vi "Aux-Inputs.vi"(8 "error in (no error)":errorcluster, 11 "Node Ptr":T2 format="%.0x") -> (0 "error out":errorcluster)   [LabVIEW 2016, in "DCM System Explorer.lvlib"]
uses:
  DCM System Explorer.lvlib
  <vilib>/NI Veristand/Custom Device API/Custom Device Item Ref.ctl
  <vilib>/Powertrain Controls/Device Drivers/DCM/Rev0/FPGA/Digital Channel.ctl
  Shared/DCM Properties.vi
  <vilib>/NI Veristand/Custom Device API/Get Item Property (String Array).vi
  <vilib>/NI Veristand/Custom Device API/Get Item Property (Double Array).vi
  <vilib>/NI Veristand/Custom Device API/Get Item Property (U16).vi
  Shared/DCM Constants and GUIDs.vi
  <vilib>/NI Veristand/Custom Device API/Set Item Property (String Array).vi
  <vilib>/NI Veristand/Custom Device API/Set Item Property (Double Array).vi
  <vilib>/NI Veristand/Custom Device API/Set Item Property (U16).vi
  <vilib>/NI VeriStand/Custom Device API/Custom Device API.lvlib
  DCM Shared.lvlib
  <vilib>/Powertrain Controls/Device Drivers/DCM/Rev0/FPGA/DCM - FPGA.lvlib
panel:
  in  "Serial Aux In 9-16":T1(ring)
  in  "Serial Aux In 1-8":T1(ring)
  in  "Digital filter [s]":sgl format="%#_2p"
  in  "Filters":sgl[](array[numeric])
  in  "_Refresh":bool
  in  "Channel Names":string[](array[string])=["", "", "", "", "", "", "", "", "", "", "", ""]
  in  "Channel Name":string
  in  "_Aux Channels":i32[](listbox) caption="Channel Summary"
  in  "Header":cluster{"Section Name":string}={"Section Name"="Aux Input Settings"}
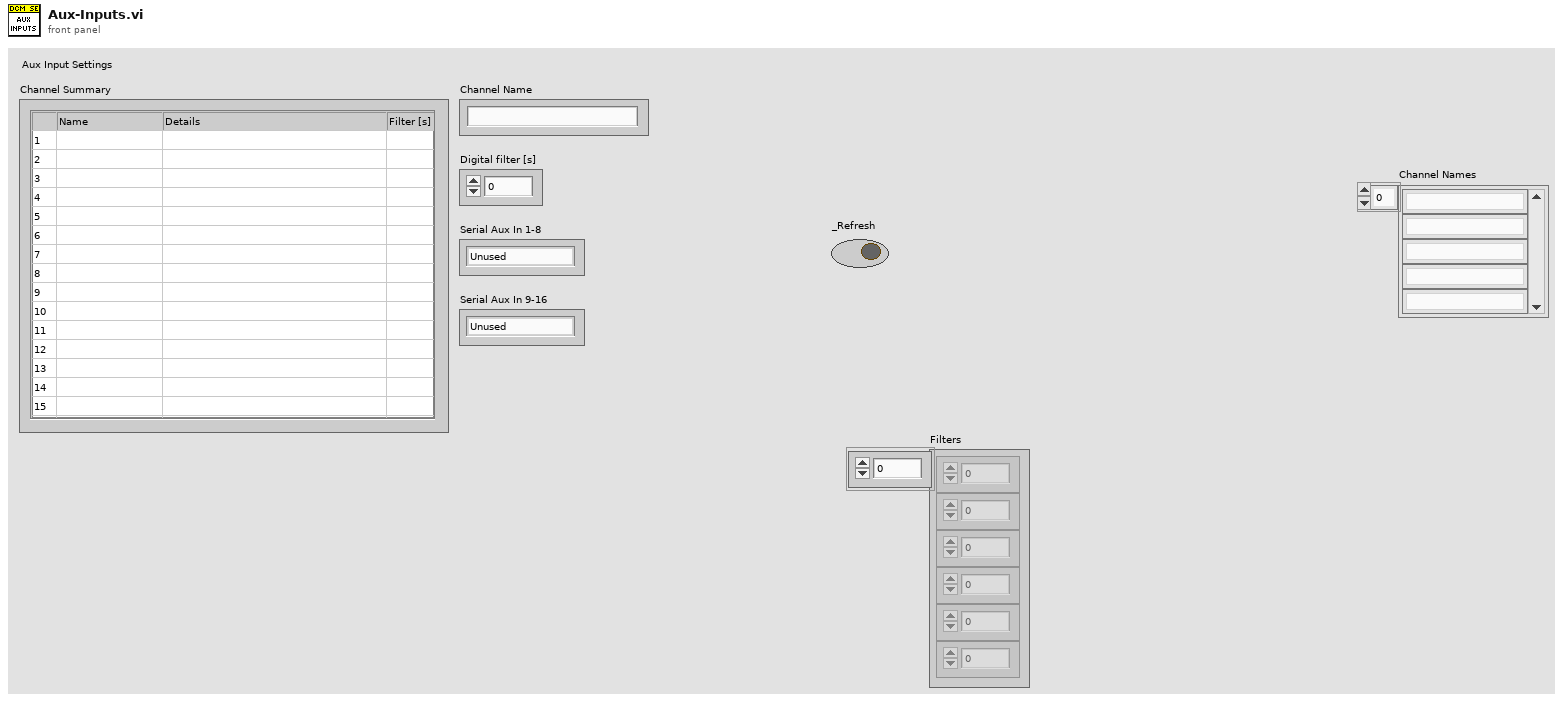
[diagram p1: front panel]
types:
  T1 = enum8{"Unused", "User OS", "Diff IO 1", "Diff IO 2", "Diff IO 3", "Diff IO 4", "Diff IO 5", "Diff IO 6", "Diff IO 7", "Diff IO 8", "Aux 1", "Aux 2", "Aux 3", "Aux 4", "Aux 5", "Aux 6", "Aux 7", "Aux 8", "Aux 9", "Aux 10", "Aux 11", "Aux 12", "Aux 13", "Aux 14", "Aux 15", "Aux 16"}
  T2 = typedef "Custom Device API.lvlib/Custom Device Item Ref.ctl" = u64
  T3 = typedef "DCM - FPGA.lvlib/Digital Channel.ctl" = enum8{"Unused", "User OS", "Diff IO 1", "Diff IO 2", "Diff IO 3", "Diff IO 4", "Diff IO 5", "Diff IO 6", "Diff IO 7", "Diff IO 8", "Aux 1", "Aux 2", "Aux 3", "Aux 4", "Aux 5", "Aux 6", "Aux 7", "Aux 8", "Aux 9", "Aux 10", "Aux 11", "Aux 12", "Aux 13", "Aux 14", "Aux 15", "Aux 16"}
  T4 = typedef "Custom Device API.lvlib/Custom Device Commands.ctl" = enum16{"Default", "Item renamed", "Shutdown", "Dynamic button pressed"}
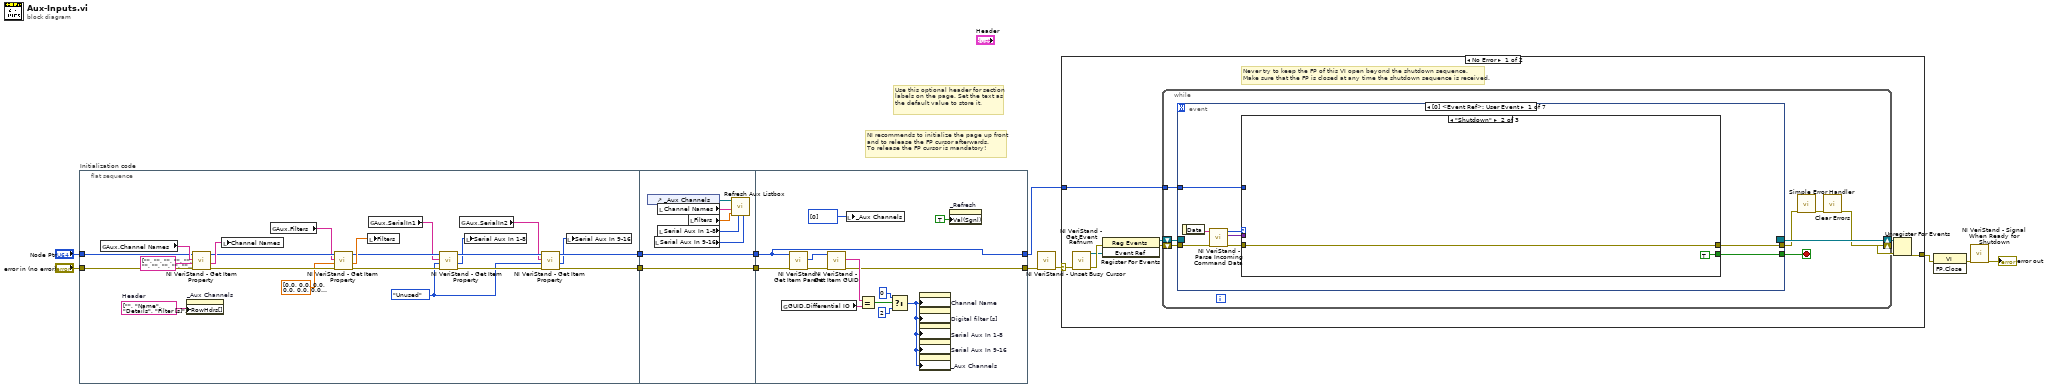
[diagram p0: block diagram]
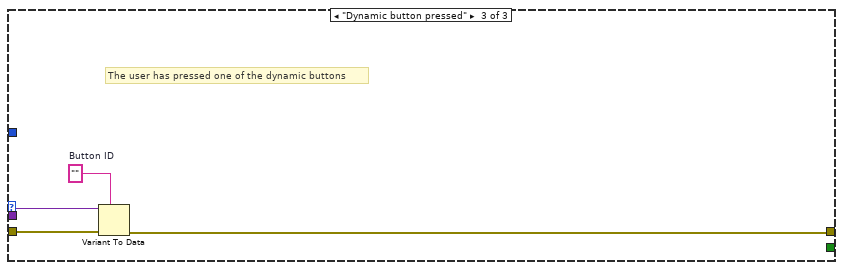
[diagram p3: hidden frame]
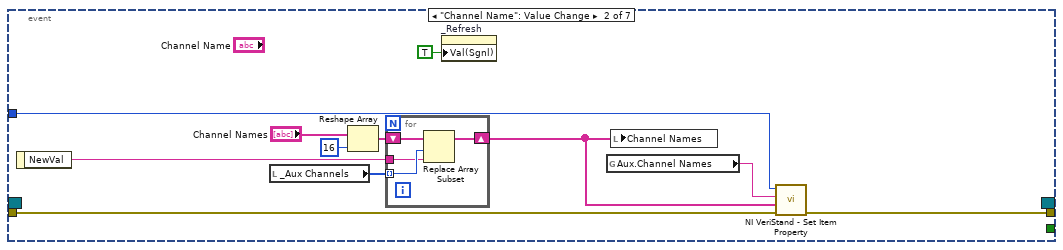
[diagram p4: hidden frame]
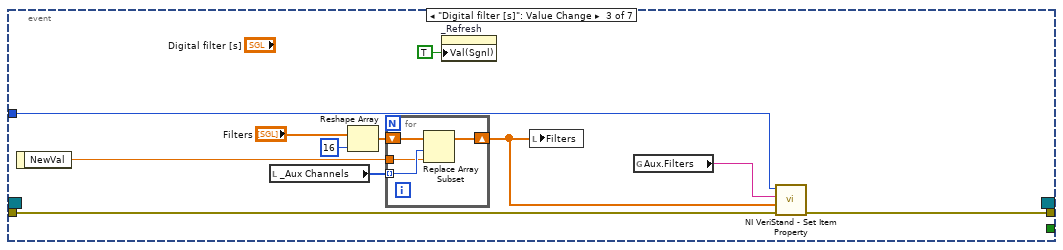
[diagram p5: hidden frame]
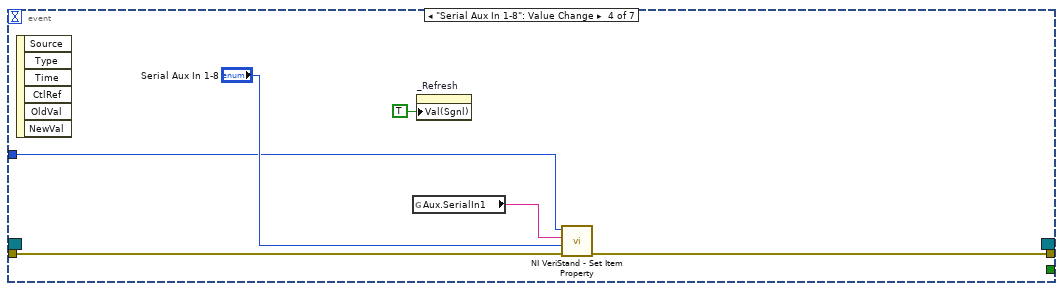
[diagram p6: hidden frame]
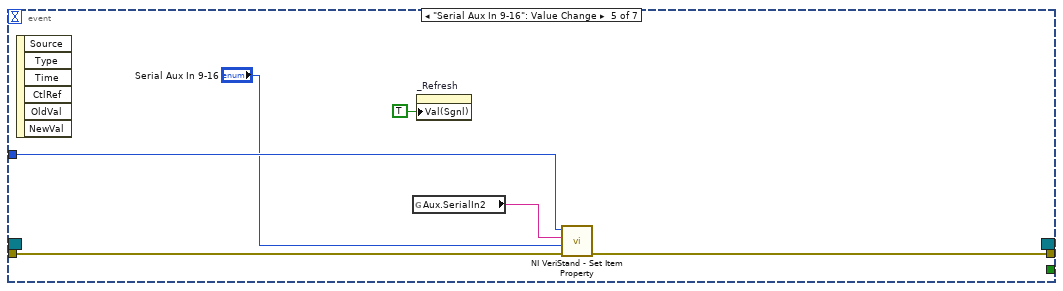
[diagram p7: hidden frame]
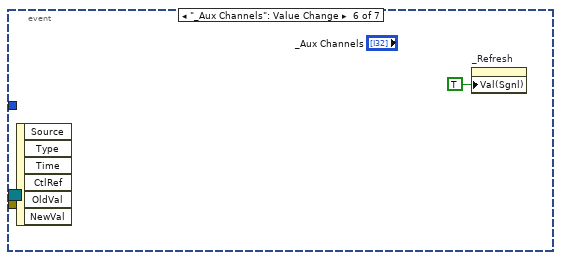
[diagram p8: hidden frame]
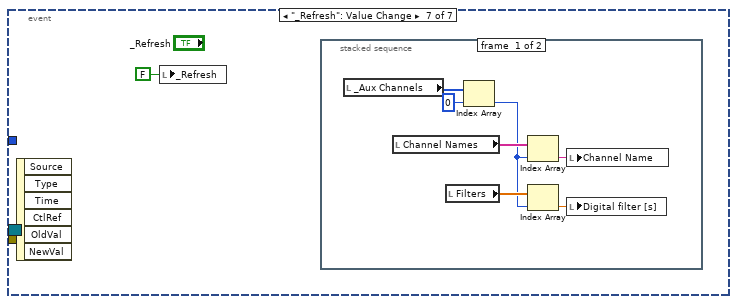
[diagram p9: hidden frame]
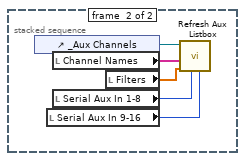
[diagram p10: hidden frame]
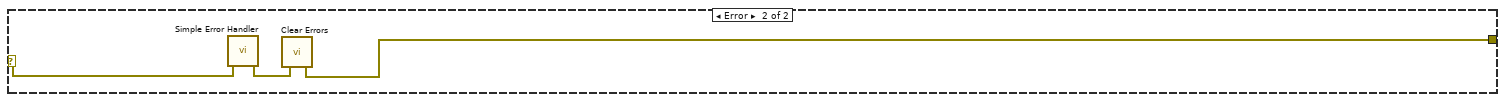
[diagram p11: hidden frame]
diagram:
  # "Use this optional header for section labels on the page. Set the text as the default value to store it."
  # "NI recommends to initialize the page up front\nand to release the FP cursor afterwards.\nTo release the FP cursor is mandatory!"
  n1 = flat-sequence "Initialization code" {
    tunnel: "Node Ptr" -> [w25]
    tunnel: "error in (no error)" -> [w24]
    tunnel: [w18] -> w12
    tunnel: [w19] -> w11
    tunnel: w12 -> [w40]
    tunnel: [w41] -> w10
    tunnel: [w40] -> w9
    tunnel: w11 -> [w41]
    tunnel: [w43] -> w1
    tunnel: [w49] -> w2
    tunnel: w10 -> [w49]
    tunnel: w9 -> [w50]
    frame #0 {
      w17 = Digital_Channel."Unused" ("Serial Aux In 1-8")
      w31 = string[] ["", "Name", "Details", "Filter [s]"]  # Header
      n2 = global read "DCM Properties.vi" "Aux.Channel Names"() -> (w34:string)
      n3 = property on="_Aux Channels" class="MCListbox (strict)"("RowHdrs[]"=w31) -> ()  [unwired: 2 in, 2 out]
      n4 = call-poly <vilib>:"NI VeriStand - Get Item Property.vi"("error in (no error)"=w24, "Default Value"=string[] ["", "", "", "", "", "", "", "", "", "", "", "", "", "", "", ""], "Property Name"=w34, "Item Ref in"=w25) -> ("error out"=w29:errorcluster, "Value"=w33:string[], "Item Ref out"=w30:T2)  [unwired: 4 in, 1 out]
      n5 = local write "Channel Names"(w33) -> ()
      n6 = global read "DCM Properties.vi" "Aux.Filters"() -> (w28:string)
      n7 = call-poly <vilib>:"NI VeriStand - Get Item Property.vi"("error in (no error)"=w29, "Default Value"=sgl[] [0.0, 0.0, 0.0, 0.0, 0.0, 0.0, 0.0, 0.0, 0.0, 0.0, 0.0, 0.0, 0.0, 0.0, 0.0, 0.0] ("Settings.Diff IO Filters [s]"), "Property Name"=w28, "Item Ref in"=w30) -> ("error out"=w22:errorcluster, "Value"=w26:dbl[], "Item Ref out"=w23:T2)  [unwired: 4 in, 1 out]
      n8 = local write "Filters"(w26) -> ()
      n9 = global read "DCM Properties.vi" "Aux.SerialIn1"() -> (w16:string)
      n10 = call-poly <vilib>:"NI VeriStand - Get Item Property.vi"("error in (no error)"=w22, "Default Value"=w17, "Property Name"=w16, "Item Ref in"=w23) -> ("error out"=w21:errorcluster, "Value"=w14:u16, "Item Ref out"=w20:T2)  [unwired: 4 in, 1 out]
      n11 = global read "DCM Properties.vi" "Aux.SerialIn2"() -> (w15:string)
      n12 = local write "Serial Aux In 1-8"(w14) -> ()
      n13 = call-poly <vilib>:"NI VeriStand - Get Item Property.vi"("error in (no error)"=w21, "Default Value"=w17, "Property Name"=w15, "Item Ref in"=w20) -> ("error out"=w18:errorcluster, "Value"=w13:u16, "Item Ref out"=w19:T2)  [unwired: 4 in, 1 out]
      n14 = local write "Serial Aux In 9-16"(w13) -> ()
    }
    frame #1 {
      n15 = control-ref of="_Aux Channels"() -> (w39:refnum<vi>)
      n16 = local read "Serial Aux In 9-16"() -> (w35:T1)
      n17 = local read "Channel Names"() -> (w38:string[])
      n18 = local read "Serial Aux In 1-8"() -> (w36:T1)
      n19 = local read "Filters"() -> (w37:sgl[])
      n20 = call "Refresh Aux Listbox.vi"("Serial Aux In 9-16"=w35, "Serial Aux In 1-8"=w36, "Filters"=w37, "Names"=w38, "MulticolumnListbox in"=w39) -> ()  [unwired: 7 in]
    }
    frame #2 {
      n21 = global read "DCM Constants and GUIDs.vi" "GUID.Differential IO"() -> (w46:string)
      n22 = call <vilib>:"NI VeriStand - Get Item Parent.vi"("error in (no error)"=w50, "Item Ref in"=w49) -> ("error out"=w44:errorcluster, "Parent Ref"=w45:T2)  [unwired: 6 in, 2 out]
      n23 = call <vilib>:"NI VeriStand - Get Item GUID.vi"("error in (no error)"=w44, "Item Ref in"=w45) -> ("error out"=w43:errorcluster, "GUID"=w47:string)  [unwired: 7 in, 1 out]
      n24 = local write "_Aux Channels"(i32[] [0] ("_DiffIO Channels")) -> ()
      n25 = Equal?(x=w47, y=w46) -> (x = y?=w42:bool)
      n26 = Select(t=0, s=w42, f=2) -> (s? t:f=w48:i32)
      n27 = property on="Channel Name" class="Str"("DisabledEnum"=w48) -> ()  [unwired: 2 in, 2 out]
      n28 = property on="Digital filter [s]" class="DigNum (strict)"("DisabledEnum"=w48) -> ()  [unwired: 2 in, 2 out]
      n29 = property on="Serial Aux In 1-8" class="Enum (strict)"("DisabledEnum"=w48) -> ()  [unwired: 2 in, 2 out]
      n30 = property on="Serial Aux In 9-16" class="Enum (strict)"("DisabledEnum"=w48) -> ()  [unwired: 2 in, 2 out]
      n31 = property on="_Aux Channels" class="MCListbox (strict)"("DisabledEnum"=w48) -> ()  [unwired: 2 in, 2 out]
      n32 = property on="_Refresh" class="Bool (strict)"("Val(Sgnl)"=TRUE ("Value (Signaling)")) -> ()  [unwired: 2 in, 2 out]
    }
  }
  n33 = call <vilib>:"NI VeriStand - Unset Busy Cursor.vi"("error in (no error)"=w1) -> ("error out"=w4:errorcluster)  [unwired: 10 out]
  n34 = case shown="No Error" w4 {
    selector: w4 -> [w56 w145]
    tunnel: [w60 w143] -> w8
    tunnel: w2 -> [w55 _]
    frame No Error {
      # "Never try to keep the FP of this VI open beyond the shutdown sequence.\nMake sure that the FP is closed at any time the shutdown sequence is received."
      n35 = call <vilib>:"NI VeriStand - Get Event Refnum.vi"("error in (no error)"=w56) -> ("error out"=w63:errorcluster, "Event Ref"=w59:refnum<user-event>)  [unwired: 9 out]
      n36 = register-events(error in=w63, w59) -> (reference out=w57:refnum<event-registration>, error out=w58:errorcluster)  [unwired: 1 in]
      n37 = while {
        shift-right: [w65] -> w61
        shift-left: w58 -> [w70]
        shift-right: [w71] -> w62
        shift-left: w57 -> [w69]
        tunnel: w55 -> [w64]
        stop <- w68 stop-if-true
        n38 = event shown="[0] <Event Ref>: User Event" {
          selector: w69 -> [_ _ _ _ _ _ _]
          dyn-events: [_ _ _ _ _ _ _] -> w71
          timeout: _ -> [_ _ _ _ _ _ _]
          tunnel: w70 -> [w79 w97 w112 w121 w127 _ _]
          tunnel: [w75 _ _ _ _ _ _] -> w68
          tunnel: [w74 w96 w111 w120 w126 _ _] -> w67
          tunnel: w64 -> [w72 w94 w109 w118 w125 _ _]
          event User Event {
            n39 = event-data() -> ("Data"=w78:string)  [unwired: 1 out]
            n40 = call <vilib>:"NI VeriStand - Parse Incoming Command Data.vi"("error in (no error)"=w79, "Incoming data"=w78) -> ("error out"=w77:errorcluster, "Outgoing data"=w73:variant, "Action"=w76:T4)  [unwired: 7 out]
            n41 = case shown="\"Shutdown\"" w76 {
              tunnel: w77 -> [w80 w81 w86]
              tunnel: [_ TRUE _] -> w75
              tunnel: [w80 w81 w83] -> w74
              tunnel: w73 -> [_ _ w85]
              tunnel: w72 -> [_ _ _]
              frame "Default", Default {
              }
              frame "Shutdown" {
              }
              frame "Dynamic button pressed" {
                w84 = ""  # Button ID
                # "The user has pressed one of the dynamic buttons"
                n42 = Variant To Data(error in=w86, type=w84, Variant=w85) -> (error out=w83:errorcluster)  [unwired: 1 out]
              }
            }
          }
          event "Channel Name": Value Change {
            n43 = event-data() -> ("NewVal"=w90:string)  [unwired: 1 out]
            n44 = local read "_Aux Channels"() -> (w91:i32[])
            n45 = Reshape Array("Channel Names", 16 ("dimension size")) -> (w93:string[])
            n46 = for {
              tunnel: w91 -> [w99] mode=indexing
              shift-right: [w100] -> w87
              shift-left: w93 -> [w101]
              tunnel: w90 -> [w98]
              n47 = Replace Array Subset(array=w101, new element=w98, index=w99) -> (w100:string[])
            }
            n48 = property on="_Refresh" class="Bool (strict)"("Val(Sgnl)"=TRUE ("Value (Signaling)")) -> ()  [unwired: 2 in, 2 out]
            n49 = global read "DCM Properties.vi" "Aux.Channel Names"() -> (w95:string)
            n50 = local write "Channel Names"(w87) -> ()
            n51 = call-poly <vilib>:"NI VeriStand - Set Item Property.vi"("error in (no error)"=w97, "Value"=w87, "Property Name"=w95, "Item Ref in"=w94) -> ("error out"=w96:errorcluster)  [unwired: 5 in, 2 out]
          }
          event "Digital filter [s]": Value Change {
            n52 = event-data() -> ("NewVal"=w105:sgl)  [unwired: 1 out]
            n53 = local read "_Aux Channels"() -> (w106:i32[])
            n54 = Reshape Array("Filters", 16 ("dimension size")) -> (w108:sgl[])
            n55 = for {
              tunnel: w106 -> [w114] mode=indexing
              shift-right: [w115] -> w102
              shift-left: w108 -> [w116]
              tunnel: w105 -> [w113]
              n56 = Replace Array Subset(array=w116, new element=w113, index=w114) -> (w115:sgl[])
            }
            n57 = property on="_Refresh" class="Bool (strict)"("Val(Sgnl)"=TRUE ("Value (Signaling)")) -> ()  [unwired: 2 in, 2 out]
            n58 = local write "Filters"(w102) -> ()
            n59 = global read "DCM Properties.vi" "Aux.Filters"() -> (w110:string)
            n60 = call-poly <vilib>:"NI VeriStand - Set Item Property.vi"("error in (no error)"=w112, "Value"=w102, "Property Name"=w110, "Item Ref in"=w109) -> ("error out"=w111:errorcluster)  [unwired: 5 in, 2 out]
          }
          event "Serial Aux In 1-8": Value Change {
            n61 = event-data() -> ()  [unwired: 7 out]
            n62 = global read "DCM Properties.vi" "Aux.SerialIn1"() -> (w122:string)
            n63 = property on="_Refresh" class="Bool (strict)"("Val(Sgnl)"=TRUE ("Value (Signaling)")) -> ()  [unwired: 2 in, 2 out]
            n64 = call-poly <vilib>:"NI VeriStand - Set Item Property.vi"("error in (no error)"=w121, "Value"="Serial Aux In 1-8", "Property Name"=w122, "Item Ref in"=w118) -> ("error out"=w120:errorcluster)  [unwired: 5 in, 2 out]
          }
          event "Serial Aux In 9-16": Value Change {
            n65 = event-data() -> ()  [unwired: 7 out]
            n66 = global read "DCM Properties.vi" "Aux.SerialIn2"() -> (w128:string)
            n67 = property on="_Refresh" class="Bool (strict)"("Val(Sgnl)"=TRUE ("Value (Signaling)")) -> ()  [unwired: 2 in, 2 out]
            n68 = call-poly <vilib>:"NI VeriStand - Set Item Property.vi"("error in (no error)"=w127, "Value"="Serial Aux In 9-16", "Property Name"=w128, "Item Ref in"=w125) -> ("error out"=w126:errorcluster)  [unwired: 5 in, 2 out]
          }
          event "_Aux Channels": Value Change {
            n69 = event-data() -> ()  [unwired: 7 out]
            n70 = property on="_Refresh" class="Bool (strict)"("Val(Sgnl)"=TRUE ("Value (Signaling)")) -> ()  [unwired: 2 in, 2 out]
          }
          event "_Refresh": Value Change {
            n71 = event-data() -> ()  [unwired: 7 out]
            n72 = local write "_Refresh"(FALSE ("_Refresh")) -> ()
            n73 = stacked-sequence {
              frame #0 {
                n74 = local read "_Aux Channels"() -> (w133:i32[])
                n75 = local read "Channel Names"() -> (w137:string[])
                n76 = local read "Filters"() -> (w135:sgl[])
                n77 = Index Array(array=w133, index=0) -> (element=w132:i32)
                n78 = Index Array(array=w137, index=w132) -> (element=w136:string)
                n79 = Index Array(array=w135, index=w132) -> (element=w134:sgl)
                n80 = local write "Channel Name"(w136) -> ()
                n81 = local write "Digital filter [s]"(w134) -> ()
              }
              frame #1 {
                n82 = control-ref of="_Aux Channels"() -> (w138:refnum<vi>)
                n83 = local read "Serial Aux In 9-16"() -> (w142:T1)
                n84 = local read "Channel Names"() -> (w139:string[])
                n85 = local read "Serial Aux In 1-8"() -> (w141:T1)
                n86 = local read "Filters"() -> (w140:sgl[])
                n87 = call "Refresh Aux Listbox.vi"("Serial Aux In 9-16"=w142, "Serial Aux In 1-8"=w141, "Filters"=w140, "Names"=w139, "MulticolumnListbox in"=w138) -> ()  [unwired: 7 in]
              }
            }
          }
        }
        n88 = call <vilib>:"Simple Error Handler.vi"("error in (no error)"=w67) -> ("error out"=w66:errorcluster)  [unwired: 1 in, 7 out]
        n89 = call <vilib>:"Clear Errors.vi"("error in (no error)"=w66) -> ("error out"=w65:errorcluster)  [unwired: 1 in, 5 out]
      }
      n90 = Unregister For Events(event registration refnum=w62, error in=w61) -> (error out=w60:errorcluster)
    }
    frame Error {
      n91 = call <vilib>:"Simple Error Handler.vi"("error in (no error)"=w145) -> ("error out"=w144:errorcluster)  [unwired: 1 in, 7 out]
      n92 = call <vilib>:"Clear Errors.vi"("error in (no error)"=w144) -> ("error out"=w143:errorcluster)  [unwired: 1 in, 5 out]
    }
  }
  n93 = invoke class="VI" method="FP.Close"(error in=w8) -> (error out=w7:errorcluster)  [unwired: 2 in, 2 out]
  n94 = call <vilib>:"NI VeriStand - Signal When Ready for Shutdown.vi"("error in (no error)"=w7) -> ("error out"=→"error out":errorcluster)  [unwired: 10 out]
